vi "1.1 Steering Controls.vi"(1 "Steering V Magnitude":i16, 2 "2.1.3 Steering V PID":T1 {"I Saturate" format="%#_14g"; "P Gain" format="%.8f"; "I Gain" format="%.8f"; "D Gain" format="%.8f"}, 3 "2.1.3 Steering PID Gains":T1 {"I Saturate" format="%#_14g"; "P Gain" format="%.8f"; "I Gain" format="%.8f"; "D Gain" format="%.8f"}, 4 "Steering Integer Setpoint":i32) -> (0 "Output":fxp<+/-,20,5> format="%.17g")   [LabVIEW 2010]
uses:
  2-Low Neurons/2.1 PID Gains Typedef.ctl
  1.0-Hindbrain Global.vi
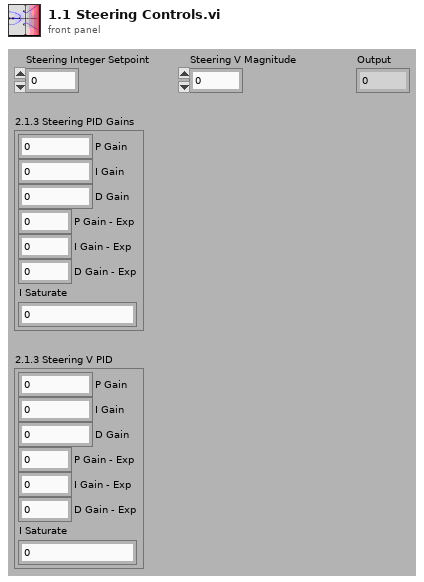
[diagram p1: front panel]
types:
  T1 = typedef "2.1 PID Gains Typedef.ctl" = cluster{"P Gain":fxp<+/-,18,1>, "I Gain":fxp<+/-,18,1>, "D Gain":fxp<+/-,18,1>, "P Gain - Exp":i8, "I Gain - Exp":i8, "D Gain - Exp":i8, "I Saturate":fxp<+/-,64,46>}
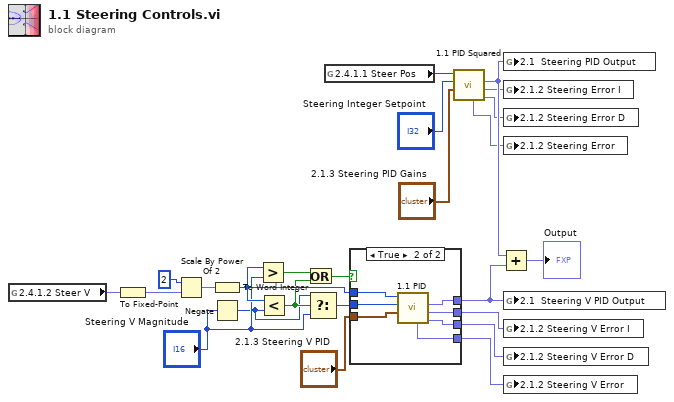
[diagram p0: block diagram]
diagram:
  n1 = global read "1.0-Hindbrain Global.vi" "2.4.1.2 Steer V"() -> (w7:fxp<+/-,10,8>)
  n2 = To Fixed-Point(number=w7) -> (fixed-point=w8:fxp<+/-,14,12>)  [unwired: 1 in]
  n3 = Scale By Power Of 2(n=2, x=w8) -> (x*2^n=w10:fxp<+/-,14,12>)
  n4 = To Word Integer(number=w10) -> (16bit integer=w18:i16)
  n5 = Negate(x="Steering V Magnitude") -> (-x=w14:i16)
  n6 = Greater?(x=w18, y="Steering V Magnitude") -> (0:w12:bool)
  n7 = Less?(x=w18, y=w14) -> (x < y?=w15:bool)
  n8 = Or(x=w12, y=w15) -> (x .or. y?=w13:bool)
  n9 = Select(t=w14, s=w15, f="Steering V Magnitude") -> (s? t:f=w17:i16)
  n10 = global read "1.0-Hindbrain Global.vi" "2.4.1.1 Steer Pos"() -> (w11:i32)
  n11 = case shown="True" w13 {
    tunnel: w17 -> [_ w31]
    tunnel: w18 -> [_ w30]
    tunnel: "2.1.3 Steering V PID" -> [_ w29]
    tunnel: [_ w28] -> w24
    tunnel: [_ w27] -> w20
    tunnel: [_ w26] -> w21
    tunnel: [_ w25] -> w22
    frame False {
    }
    frame True {
      n12 = call "1.1 PID.vi"("2.1 PID Gains"=w29, "Setpoint"=w31, "Encoder Value"=w30) -> ("D Error"=w26:fxp<+/-,18,1>, "I Error"=w25:fxp<+/-,64,46>, "Analog Output"=w28:fxp<+/-,20,5>, "Error"=w27:fxp<+/-,18,1>)  [unwired: 5 in]
    }
  }
  n13 = call "1.1 PID Squared .vi"("2.1 PID Gains"="2.1.3 Steering PID Gains", "Setpoint"="Steering Integer Setpoint", "Encoder Value"=w11) -> ("D Error"=w4:fxp<+/-,18,1>, "I Error"=w5:fxp<+/-,64,46>, "Analog Output"=w6:fxp<+/-,20,5>, "Error"=w3:fxp<+/-,18,1>)  [unwired: 5 in]
  n14 = Add(x=w6, y=w24) -> (x+y=→"Output":fxp<+/-,20,5>)
  n15 = global write "1.0-Hindbrain Global.vi" "2.1  Steering PID Output"(w6) -> ()
  n16 = global write "1.0-Hindbrain Global.vi" "2.1.2 Steering Error I"(w5) -> ()
  n17 = global write "1.0-Hindbrain Global.vi" "2.1.2 Steering Error D"(w4) -> ()
  n18 = global write "1.0-Hindbrain Global.vi" "2.1.2 Steering Error"(w3) -> ()
  n19 = global write "1.0-Hindbrain Global.vi" "2.1  Steering V PID Output"(w24) -> ()
  n20 = global write "1.0-Hindbrain Global.vi" "2.1.2 Steering V Error I"(w22) -> ()
  n21 = global write "1.0-Hindbrain Global.vi" "2.1.2 Steering V Error D"(w21) -> ()
  n22 = global write "1.0-Hindbrain Global.vi" "2.1.2 Steering V Error"(w20) -> ()
